vi "Record_GPS_log.vi"() -> ()   [LabVIEW 2019]
uses:
  Ctrl/gps-232.ctl
panel:
  out "loop i":i32
  out "heading_val":bool
  out "mode validate":bool
  out "heading data":string
  out "lat long":string
  in  "save":bool
  out "XY 그래프":cluster{"X":dbl, "Y":dbl}[](graph)
  out "경도":string="126.72082016226"
  out "위도":string="37.37012814476"
  out "utm-1":cluster{dbl, dbl}={530126.7583503594, 175270.68061157822} {"?" format="%.2f"; "?" format="%.2g"}
  out "wgs84-1":cluster{dbl, dbl}={126.72082016226, 37.37012814476}
  out "heading 1":dbl(graph)=228.865081787
  out "heading str":string="228.865081787"
  out "serial read buf":u32
  out "read data":string
  in  "정지":bool
  in  "baud rate gps":u32=115200
  # "GNSS test"
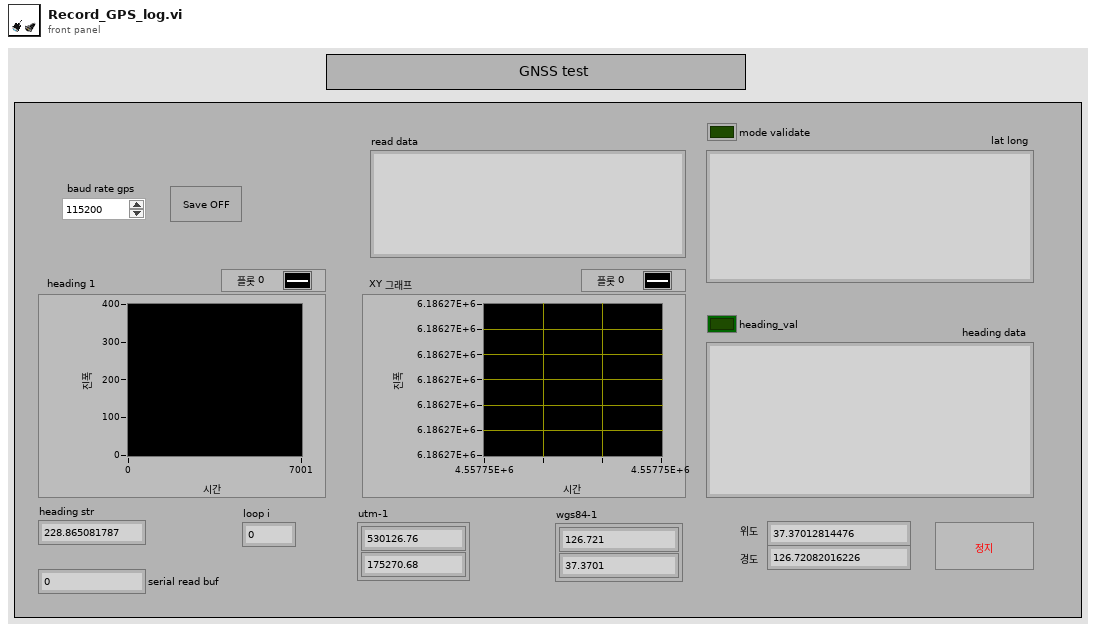
[diagram p1: front panel]
types:
  T1 = typedef "gps-232.ctl" = enum16{"ini", "timing set", "read", "write", "close"}
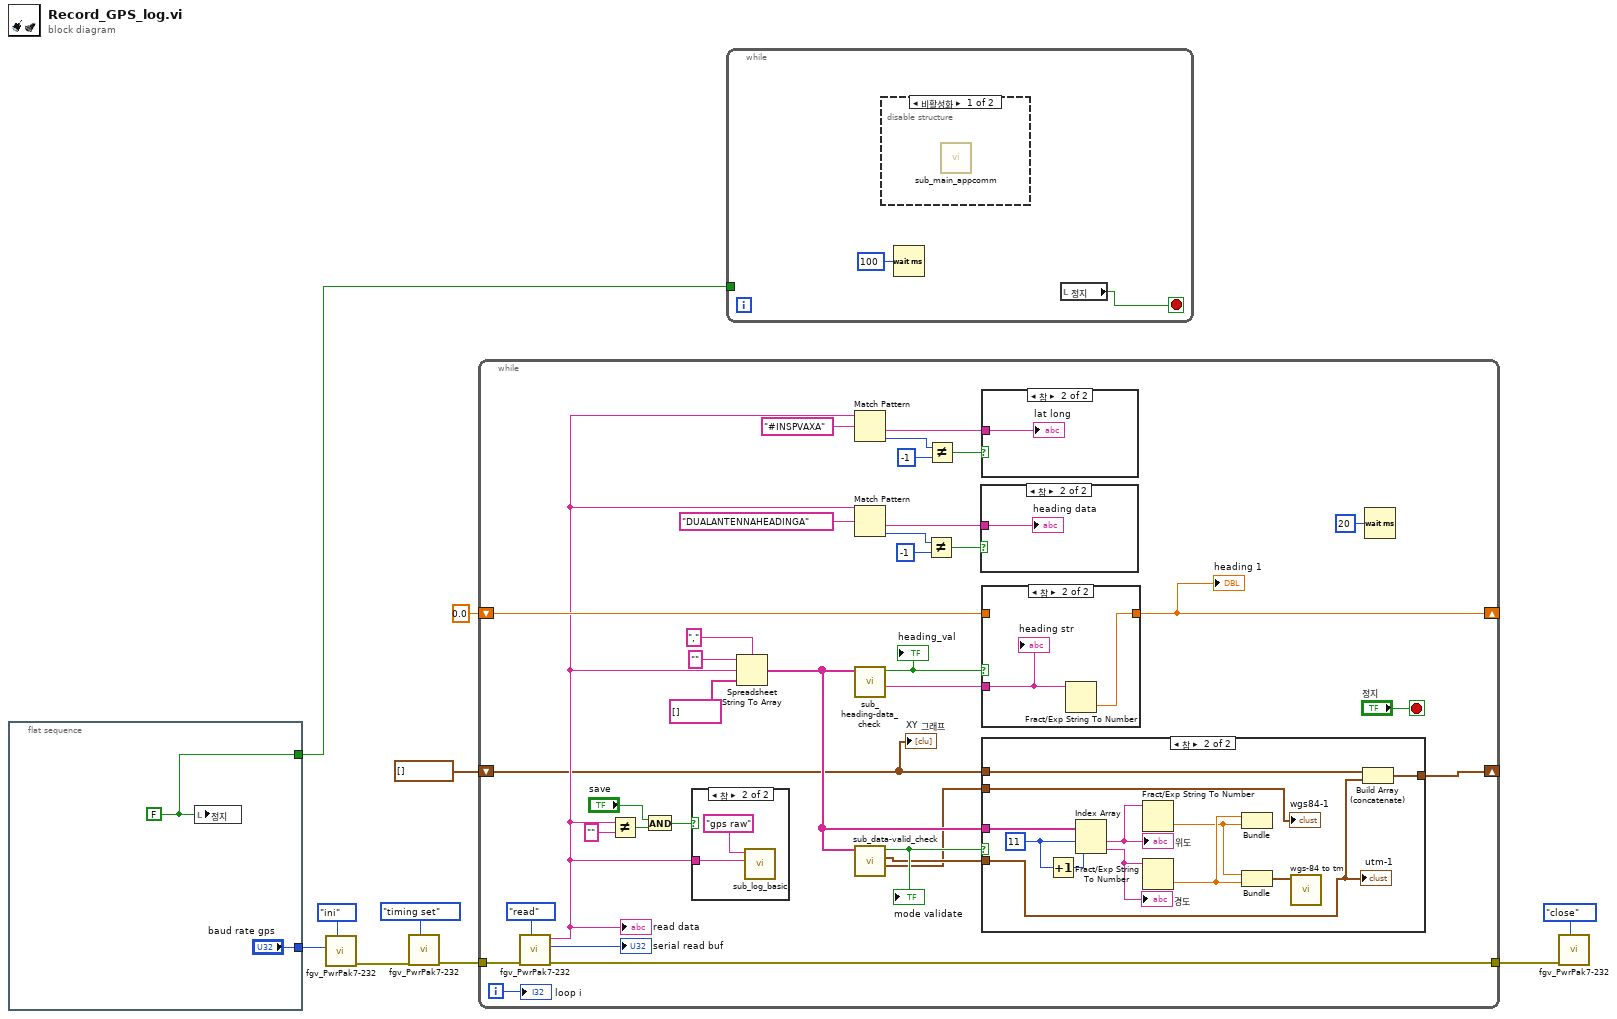
[diagram p0: block diagram]
diagram:
  n1 = flat-sequence {
    tunnel: ["baud rate gps"] -> w10
    tunnel: [w11] -> w1
    frame #0 {
      w11 = FALSE ("정지")
      n2 = local write "정지"(w11) -> ()
    }
  }
  n3 = call "fgv_PwrPak7-232.vi"("cmd"=gps-232."ini", "baud rate"=w10) -> ("error out"=w9:errorcluster)  [unwired: 6 in, 3 out]
  n4 = call "fgv_PwrPak7-232.vi"("cmd"=gps-232."timing set", "error in"=w9) -> ("error out"=w6:errorcluster)  [unwired: 6 in, 3 out]
  n5 = while {
    tunnel: w6 -> [w45]
    tunnel: [w44] -> w4
    shift-right: [w37] -> _
    shift-left: 0.0 -> [w38]
    shift-right: [w33] -> _
    shift-left: cluster{"Y(E)":dbl, "X(N)":dbl}[] [] -> [w16]
    i -> [w15]
    stop <- "정지" stop-if-true
    n6 = call "fgv_PwrPak7-232.vi"("cmd"=gps-232."read", "error in"=w45) -> ("error out"=w44:errorcluster, "buff"=→"serial read buf":u32, "read data"=w21:string)  [unwired: 6 in, 1 out]
    "read data" <- w21
    n7 = Not Equal?(x=w21, y="") -> (x != y?=w19:bool)
    n8 = And(x="save", y=w19) -> (x .and. y?=w17:bool)
    n9 = case shown="참" w17 {
      tunnel: w21 -> [_ w50]
      frame False {
      }
      frame True {
        n10 = call "sub_log_basic.vi"("desc"=w50, "Title"="gps raw") -> ()  [unwired: 9 in, 1 out]
      }
    }
    n11 = Spreadsheet String To Array(delimiter (Tab)="," ("구분 문자 (탭)"), format string="" ("포맷 문자열"), spreadsheet string=w21, array type (2D Dbl)=string[] []) -> (array=w36:string[])
    n12 = Match Pattern(string=w21, regular expression="#INSPVAXA" ("정규식")) -> (after substring=w28:string, offset past match=w31:i32)  [unwired: 1 in, 2 out]
    n13 = Match Pattern(string=w21, regular expression="DUALANTENNAHEADINGA" ("정규식")) -> (after substring=w23:string, offset past match=w26:i32)  [unwired: 1 in, 2 out]
    n14 = call "sub_heading-data_check.vi"("gps received data-arr"=w36) -> ("heading_str"=w34:string, "heading_check"=w35:bool)  [unwired: 8 in, 1 out]
    "heading_val" <- w35
    n15 = call "sub_data-valid_check.vi"("gps receive parsing array"=w36) -> ("wgs84-1"=w13:cluster{dbl, dbl}, "utm-1"=w14:cluster{dbl, dbl}, "mode check"=w22:bool)  [unwired: 8 in]
    "mode validate" <- w22
    n16 = Not Equal?(x=w26, y=-1) -> (x != y?=w24:bool)
    n17 = Not Equal?(x=w31, y=-1) -> (x != y?=w29:bool)
    n18 = case shown="참" w24 {
      tunnel: w23 -> [_ w48]
      frame False {
      }
      frame True {
        "heading data" <- w48
      }
    }
    n19 = case shown="참" w29 {
      tunnel: w28 -> [_ w49]
      frame False {
      }
      frame True {
        "lat long" <- w49
      }
    }
    n20 = case shown="참" w35 {
      tunnel: [w65 w67] -> w37
      tunnel: w38 -> [w65 _]
      tunnel: w34 -> [_ w66]
      frame False {
      }
      frame True {
        n21 = Fract/Exp String To Number(string=w66) -> (number=w67:dbl)  [unwired: 3 in, 1 out]
        "heading str" <- w66
      }
    }
    "heading 1" <- w37
    n22 = case shown="참" w22 {
      tunnel: w36 -> [_ w60]
      tunnel: [w52 w58] -> w33
      tunnel: w16 -> [w52 w57]
      tunnel: w14 -> [_ w54]
      tunnel: w13 -> [_ w53]
      frame False {
      }
      frame True {
        w55 = 11 ("index")
        n23 = Increment(x=w55) -> (x+1=w56:i32)
        n24 = Index Array(array=w60, index #1=w55, index #2=w56) -> (element #1=w64:string, element #2=w59:string)
        "위도" <- w64
        "경도" <- w59
        n25 = Fract/Exp String To Number(string=w64) -> (number=w62:dbl)  [unwired: 3 in, 1 out]
        n26 = Fract/Exp String To Number(string=w59) -> (number=w63:dbl)  [unwired: 3 in, 1 out]
        n27 = Bundle(w63, w62) -> ()  [unwired: 1 in, 1 out]
        n28 = Bundle(w62, w63) -> (w61:cluster{dbl, dbl})  [unwired: 1 in]
        n29 = call "wgs-84 to tm.vi"("in_lon-lat"=w61) -> ()  [unwired: 10 in, 1 out]
        n30 = Build Array (concatenate)(w57, w54) -> (w58:cluster{"Y(E)":dbl, "X(N)":dbl}[])
        "wgs84-1" <- w53
        "utm-1" <- w54
      }
    }
    n31 = Wait (ms)(milliseconds to wait=u32 20 ("대기 시간 (ms)")) -> ()  [unwired: 1 out]
    "XY 그래프" <- w16
    "loop i" <- w15
  }
  n32 = while {
    tunnel: w1 -> [_]
    stop <- w69 stop-if-true
    n33 = disable-structure shown="비활성화" {
      frame Disabled {
        n34 = call "sub_main_appcomm.vi"() -> ()  [unwired: 11 in, 1 out]
      }
      frame Enabled {
      }
    }
    n35 = Wait (ms)(milliseconds to wait=u32 100 ("대기 시간 (ms)")) -> ()  [unwired: 1 out]
    n36 = local read "정지"() -> (w69:bool)
  }
  n37 = call "fgv_PwrPak7-232.vi"("cmd"=gps-232."close", "error in"=w4) -> ()  [unwired: 6 in, 4 out]
